vi "Strip Topic Name.vi"(2 "Topic":string) -> (6 "Topic name":string)   [LabVIEW 2018]
doc: "Strips the topic name from the path. Assumes that name is third item in path."
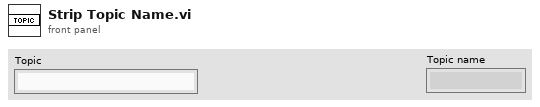
[diagram p1: front panel]
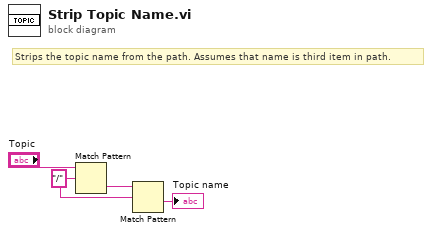
[diagram p0: block diagram]
diagram:
  w2 = "/" ("regular expression")
  # "Strips the topic name from the path. Assumes that name is third item in path."
  n1 = Match Pattern(string="Topic", regular expression=w2) -> (after substring=w3:string)  [unwired: 1 in, 3 out]
  n2 = Match Pattern(string=w3, regular expression=w2) -> (after substring=→"Topic name":string)  [unwired: 1 in, 3 out]
